vi "GW_PEPS_CmdStr.vi"(1 "GW_PEPS信息":T1 {"PEPS电源模式" items=["OFF", "ACC", "ON", "Reserved", "START", "Reserved", "Reserved", "Reserved"]; "PEPS电源模式有效指示" items=["Not available", "Invalid", "Valid", "Reserved"]}) -> (0 "CmdStr":string)   [LabVIEW 2013]
uses:
  GW_PEPS_2FC.ctl
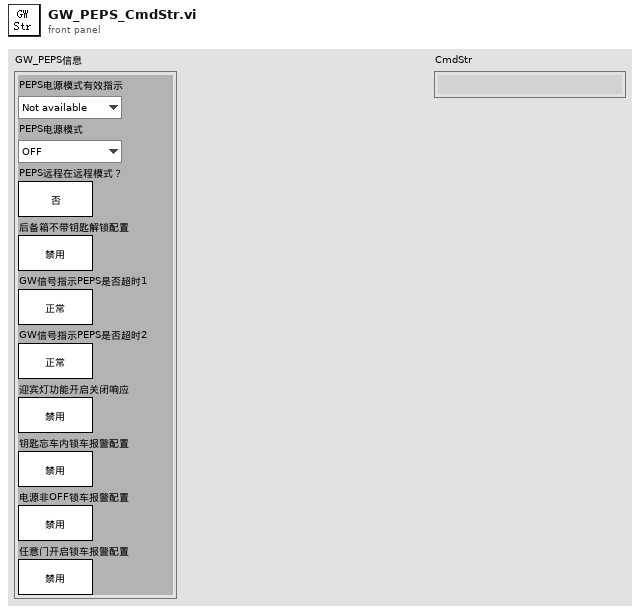
[diagram p1: front panel]
types:
  T1 = typedef "GW_PEPS_2FC.ctl" = cluster{"PEPS电源模式有效指示":u16, "PEPS电源模式":u16, "PEPS远程在远程模式？":bool, "后备箱不带钥匙解锁配置":bool, "GW信号指示PEPS是否超时1":bool, "GW信号指示PEPS是否超时2":bool, "迎宾灯功能开启关闭响应":bool, "钥匙忘车内锁车报警配置":bool, "电源非OFF锁车报警配置":bool, "任意门开启锁车报警配置":bool}
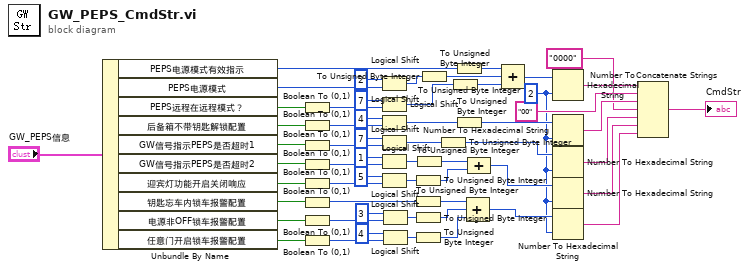
[diagram p0: block diagram]
diagram:
  w3 = 2
  n1 = Unbundle By Name("GW_PEPS信息") -> ("PEPS电源模式有效指示"=w53:u16, "PEPS电源模式"=w56:u16, "PEPS远程在远程模式？"=w50:bool, "后备箱不带钥匙解锁配置"=w41:bool, "GW信号指示PEPS是否超时1"=w33:bool, "GW信号指示PEPS是否超时2"=w26:bool, "迎宾灯功能开启关闭响应"=w22:bool, "钥匙忘车内锁车报警配置"=w11:bool, "电源非OFF锁车报警配置"=w16:bool, "任意门开启锁车报警配置"=w8:bool)
  n2 = Boolean To (0,1)(Boolean=w50) -> (0, 1=w49:i16)
  n3 = Boolean To (0,1)(Boolean=w41) -> (0, 1=w43:i16)
  n4 = Boolean To (0,1)(Boolean=w33) -> (0, 1=w34:i16)
  n5 = Boolean To (0,1)(Boolean=w26) -> (0, 1=w29:i16)
  n6 = Boolean To (0,1)(Boolean=w22) -> (0, 1=w23:i16)
  n7 = Boolean To (0,1)(Boolean=w11) -> (0, 1=w9:i16)
  n8 = Boolean To (0,1)(Boolean=w16) -> (0, 1=w17:i16)
  n9 = Boolean To (0,1)(Boolean=w8) -> (0, 1=w15:i16)
  n10 = Logical Shift(y=2, x=w56) -> (x << y=w52:u16)
  n11 = Logical Shift(y=7, x=w49) -> (x << y=w51:i16)
  n12 = Logical Shift(y=4, x=w43) -> (x << y=w39:i16)
  n13 = Logical Shift(y=7, x=w34) -> (x << y=w35:i16)
  n14 = Logical Shift(y=1, x=w29) -> (x << y=w28:i16)
  n15 = Logical Shift(y=5, x=w23) -> (x << y=w20:i16)
  n16 = Logical Shift(y=3, x=w17) -> (x << y=w13:i16)
  n17 = Logical Shift(y=4, x=w15) -> (x << y=w12:i16)
  n18 = To Unsigned Byte Integer(number=w20) -> (unsigned 8bit integer=w10:u8)
  n19 = To Unsigned Byte Integer(number=w9) -> (unsigned 8bit integer=w7:u8)
  n20 = To Unsigned Byte Integer(number=w13) -> (unsigned 8bit integer=w6:u8)
  n21 = To Unsigned Byte Integer(number=w12) -> (unsigned 8bit integer=w5:u8)
  n22 = To Unsigned Byte Integer(number=w28) -> (unsigned 8bit integer=w24:u8)
  n23 = To Unsigned Byte Integer(number=w52) -> (unsigned 8bit integer=w47:u8)
  n24 = To Unsigned Byte Integer(number=w35) -> (unsigned 8bit integer=w31:u8)
  n25 = To Unsigned Byte Integer(number=w51) -> (unsigned 8bit integer=w40:u8)
  n26 = To Unsigned Byte Integer(number=w53) -> (unsigned 8bit integer=w48:u8)
  n27 = To Unsigned Byte Integer(number=w39) -> (unsigned 8bit integer=w38:u8)
  n28 = Compound Arithmetic op=ADD(w7, w6, w5) -> (w4:u8)
  n29 = Compound Arithmetic op=ADD(w24, w10) -> (w19:u8)
  n30 = Compound Arithmetic op=ADD(w48, w47, w40) -> (w46:u8)
  n31 = Number To Hexadecimal String(1:w3, 2:w46) -> (0:w45:string)
  n32 = Number To Hexadecimal String(1:w3, 2:w38) -> (0:w37:string)
  n33 = Number To Hexadecimal String(1:w3, 2:w31) -> (0:w30:string)
  n34 = Number To Hexadecimal String(1:w3, 2:w19) -> (0:w25:string)
  n35 = Number To Hexadecimal String(1:w3, 2:w4) -> (0:w2:string)
  n36 = Concatenate Strings(w45, "00", w37, "0000", w30, w25, w2) -> (→"CmdStr":string)
